vi "Get CT Offsets.vi"(8 "error in":errorcluster, 11 "Path":path) -> (0 "error out":errorcluster, 3 "CT Offsets":fxp<+,24,6>[](array[numeric]))   [LabVIEW 2019]
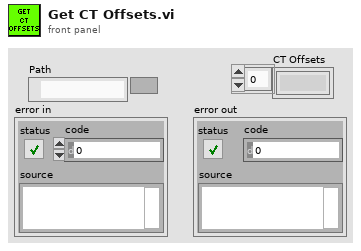
[diagram p1: front panel]
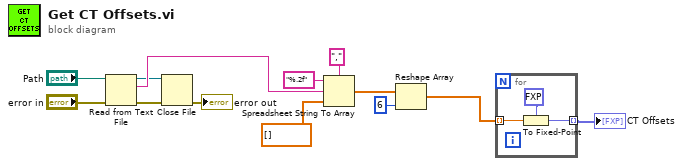
[diagram p0: block diagram]
diagram:
  n1 = Read from Text File(file (use dialog)="Path", error in="error in") -> (refnum out=w12:refnum<file>, text=w13:string, error out=w11:errorcluster)  [unwired: 2 in, 1 out]
  n2 = Close File(refnum=w12, error in=w11) -> (error out=→"error out":errorcluster)  [unwired: 1 out]
  n3 = Spreadsheet String To Array(delimiter (Tab)=",", format string="%.2f", spreadsheet string=w13, array type (2D Dbl)=dbl[] []) -> (array=w4:dbl[])
  n4 = Reshape Array(w4, 6 ("dimension size")) -> (w9:dbl[])
  n5 = for {
    tunnel: w9 -> [w16] mode=indexing
    tunnel: [w14] -> w8 mode=indexing
    n6 = To Fixed-Point(fixed-point type=fxp<+,24,6> 0.0 ("RMS"), number=w16) -> (fixed-point=w14:fxp<+,24,6>)
  }
  "CT Offsets" <- w8
